vi "Analog_Output_8Channels_W20I5.vi"(1 "Values":fxp<+/-,20,5>[](array[numeric])=[0.0, 0.0, 0.0, 0.0, 0.0, 0.0, 0.0, 0.0], 2 "IO":T1={"AO 0"="Connector1/AO0", "AO 1"="Connector1/AO0", "AO 2"="Connector1/AO0", "AO 3"="Connector1/AO0", "AO 4"="Connector1/AO0", "AO 5"="Connector1/AO0", "AO 6"="Connector1/AO0", "AO 7"="Connector1/AO0"}) -> ()   [LabVIEW 2015, in "FPGA Wizard Templates.lvlib"]
uses:
  FPGA Wizard Templates.lvlib
  <vilib>/rvi/eio/common/nirviEmuTemplateMethod_errors.vi
  <vilib>/eio/EIONode/EIONode.xnode
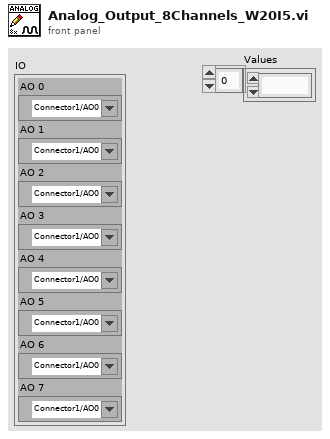
[diagram p1: front panel]
types:
  T1 = cluster{"AO 0":refnum<k21>, "AO 1":refnum<k21>, "AO 2":refnum<k21>, "AO 3":refnum<k21>, "AO 4":refnum<k21>, "AO 5":refnum<k21>, "AO 6":refnum<k21>, "AO 7":refnum<k21>}
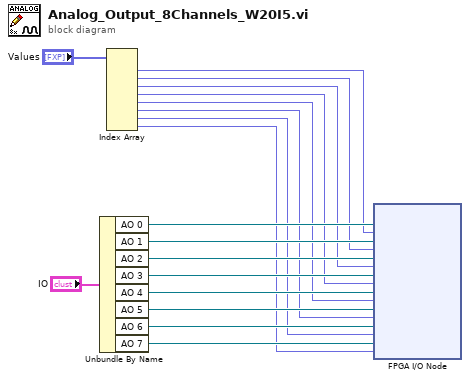
[diagram p0: block diagram]
diagram:
  n1 = Unbundle By Name("IO") -> ("AO 0"=w17:refnum<k21>, "AO 1"=w16:refnum<k21>, "AO 2"=w15:refnum<k21>, "AO 3"=w14:refnum<k21>, "AO 4"=w13:refnum<k21>, "AO 5"=w12:refnum<k21>, "AO 6"=w11:refnum<k21>, "AO 7"=w10:refnum<k21>)
  n2 = Index Array(array="Values") -> (element #1=w8:fxp<+/-,20,5>, element #2=w7:fxp<+/-,20,5>, element #3=w6:fxp<+/-,20,5>, element #4=w5:fxp<+/-,20,5>, element #5=w4:fxp<+/-,20,5>, element #6=w3:fxp<+/-,20,5>, element #7=w2:fxp<+/-,20,5>, element #8=w1:fxp<+/-,20,5>)  [unwired: 8 in]
  n3 = xnode "FPGA I/O Node"("I/O Item"=w8, "FPGA I/O In"=w17, "I/O Item"=w7, "FPGA I/O In"=w16, "I/O Item"=w6, "FPGA I/O In"=w15, "I/O Item"=w5, "FPGA I/O In"=w14, "I/O Item"=w4, "FPGA I/O In"=w13, "I/O Item"=w3, "FPGA I/O In"=w12, "I/O Item"=w2, "FPGA I/O In"=w11, "I/O Item"=w1, "FPGA I/O In"=w10) -> ()  [unwired: 8 out]
